vi "Read amplitude.vi"(8 "error in (no error)":errorcluster, 11 "Wfm_PulseMeasurement in":refnum<class "Wfm_PulseMeasurement.lvclass">) -> (0 "error out":errorcluster, 1 "pulse duration":dbl, 2 "period":dbl format="%.2g", 3 "Wfm_PulseMeasurement out":refnum<class "Wfm_PulseMeasurement.lvclass">, 4 "duty cycle":dbl, 6 "measurement info":T1)   [LabVIEW 2012, in "MyApp.lvlib" / "Wfm_PulseMeasurement.lvclass"]
uses:
  Wfm_PulseMeasurement.lvclass
  Wfm_PulseMeasurement.lvclass/Wfm_PulseMeasurement.ctl
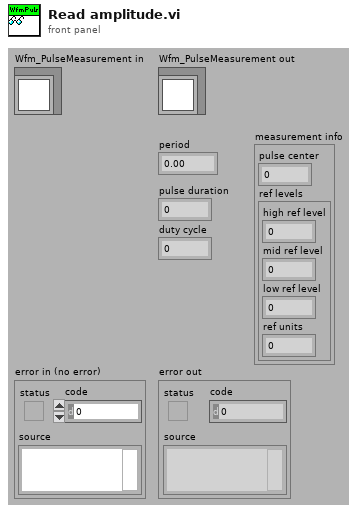
[diagram p1: front panel]
types:
  T1 = cluster{"pulse center":dbl, "ref levels":cluster{"high ref level":dbl, "mid ref level":dbl, "low ref level":dbl, "ref units":u16}}
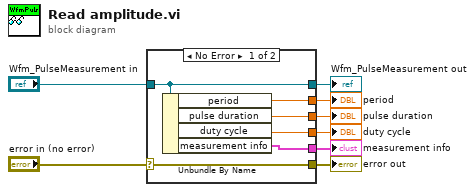
[diagram p0: block diagram]
diagram:
  n1 = case shown="No Error" "error in (no error)" {
    selector: "error in (no error)" -> [w14 w15]
    tunnel: [w14 w15] -> w7
    tunnel: [w13 w16] -> w5
    tunnel: "Wfm_PulseMeasurement in" -> [w13 w16]
    tunnel: [w12 _] -> w4
    tunnel: [w11 _] -> w3
    tunnel: [w10 _] -> w2
    tunnel: [w9 _] -> w1
    frame No Error {
      n2 = Unbundle By Name(w13) -> ("period"=w12:dbl, "pulse duration"=w11:dbl, "duty cycle"=w10:dbl, "measurement info"=w9:T1)
    }
    frame Error {
    }
  }
  "error out" <- w7
  "Wfm_PulseMeasurement out" <- w5
  "duty cycle" <- w2
  "measurement info" <- w1
  "period" <- w4
  "pulse duration" <- w3
